vi "624WPI_DashboardGetInfo.vi"(7 "Vision":u16(ring) items=["Camera Off", "USB Camera SW", "USB Camera HW", "IP Camera"], 8 "Binding Refnum":refnum<notifier>, 9 "Window Mode Notifier":refnum<notifier>, 11 "TCP Cnx":refnum<k5>) -> (0 "Power and Errors":T2, 1 "Robot Metrics":T3, 2 "Status Info":T5, 3 "Control Info":T4 {"Team Station" items=["Red 1", "Red 2", "Red 3", "Blue 1", "Blue 2", "Blue 3"]}, 4 "Robot Mode":T1(ring), 5 "Process?":bool, 6 "Custom Dashboard Data":string)   [LabVIEW 2017]
uses:
  Dashboard Hijack Data.ctl
  <vilib>/Rock Robotics/WPI/Dashboard/WPI_DashboardLogging Global.vi
panel:
  out "port":u16
  # "CAN Metrics\nJS HID Outputs\nFree Mem"
  # "Need to merge in TCP info too"
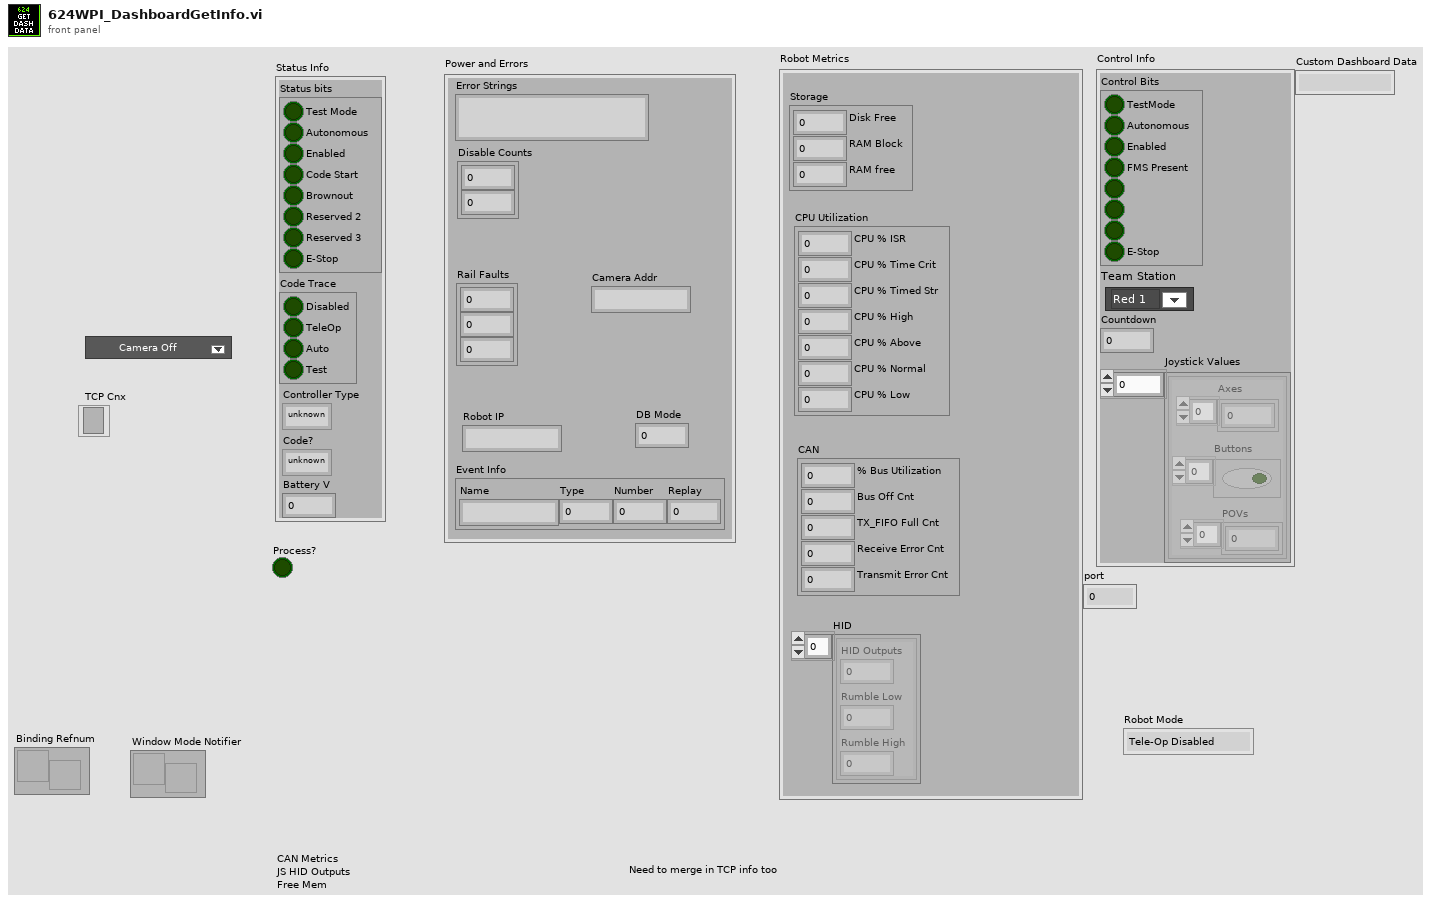
[diagram p1: front panel]
types:
  T1 = enum8{"Tele-Op Disabled", "Tele-Op Enabled", "Auto Disabled", "Auto Enabled", "Test Disabled", "Test Enabled", "Disconnected", "No Code", "E-Stop"}
  T2 = cluster{"Error Strings":string, "Disable Counts":cluster{u16, u16}, "Rail Faults":cluster{u16, u16, u16}, "Robot IP":string, "DB Mode":u8, "Event Info":cluster{"Name":string, "Type":u8, "Number":u16, "Replay":u8}, "Camera Addr":string}
  T3 = cluster{"Storage":cluster{"Disk Free":u64, "RAM Block":u32, "RAM free":u32}, "CPU Utilization":cluster{"CPU % ISR":sgl, "CPU % Time Crit":sgl, "CPU % Timed Str":sgl, "CPU % High":sgl, "CPU % Above":sgl, "CPU % Normal":sgl, "CPU % Low":sgl}, "CAN":cluster{"% Bus Utilization":sgl, "Bus Off Cnt":u32, "TX_FIFO Full Cnt":u32, "Receive Error Cnt":u8, "Transmit Error Cnt":u8}, "HID":cluster{"HID Outputs":u32, "Rumble Low":u16, "Rumble High":u16}[]}
  T4 = cluster{"Control Bits":cluster{"TestMode":bool, "Autonomous":bool, "Enabled":bool, "FMS Present":bool, bool, bool, bool, "E-Stop":bool}, "Team Station ":u8, "Countdown":sgl, "Joystick Values":cluster{"Axes":dbl[], "Buttons":bool[], "POVs":i16[]}[]}
  T5 = cluster{"Status bits":cluster{"Test Mode":bool, "Autonomous":bool, "Enabled":bool, "Code Start":bool, "Brownout":bool, "Reserved 2":bool, "Reserved 3":bool, "E-Stop":bool}, "Code Trace":cluster{"Disabled":bool, "TeleOp":bool, "Auto":bool, "Test":bool}, "Controller Type":enum16{"unknown", "cRIO", "roboRio"}, "Code?":enum16{"unknown", "noCode", "code"}, "Battery V":dbl}
  T6 = typedef "Dashboard Hijack Data.ctl" = cluster{"UDP Status string":string, "Extra data string":string}
  T7 = cluster{"TestMode":bool, "Autonomous":bool, "Enabled":bool, "FMS Present":bool, bool, bool, bool, "E-Stop":bool}
  T8 = enum16{"Standard", "Buffered", "CRLF", "Immediate"}
  T9 = cluster{"UDP Status":string, "TCP":string, "UDP Control":string}
  T10 = cluster{cluster{"Disk Free":u64, "RAM Block":u32, "RAM free":u32}, cluster{"CPU Load ISR":sgl, "CPU Load Time Critical Pr":sgl, "CPU Load Timed Str Pr":sgl, "CPU Load High Pr":sgl, "CPU Load Above Normal Pr":sgl, "CPU Load Normal Pr":sgl, "CPU Load Low Pr":sgl}, cluster{"% Bus Utilization":sgl, "Bus Off Cnt":u32, "TX_FIFO Full Cnt":u32, "Receive Error Cnt":u8, "Transmit Error Cnt":u8}, cluster{"HID Outputs":u32, "Rumble Low":u16, "Rumble High":u16}[]}
  T11 = cluster{"Status":cluster{"Test Mode":bool, "Autonomous":bool, "Enabled":bool, "Code Start":bool, "Brownout":bool, "Reserved 2":bool, "Reserved 3":bool, "E-Stop":bool}, cluster{bool, bool, bool, bool}, "ctrl":enum16{"unknown", "cRIO", "roboRio"}, "code?":enum16{"unknown", "noCode", "code"}, dbl}
  T12 = cluster{"Boolean array":cluster{"Boolean array[0]":bool, "Boolean array[1]":bool, "Boolean array[2]":bool, "Boolean array[3]":bool, "Boolean array[4]":bool, "Boolean array[5]":bool, "Boolean array[6]":bool, "Boolean array[7]":bool}, u8, "Countdown":sgl, cluster{dbl[], bool[], i16[]}[]}
  T13 = cluster{"Boolean array[0]":bool, "Boolean array[1]":bool, "Boolean array[2]":bool, "Boolean array[3]":bool, "Boolean array[4]":bool, "Boolean array[5]":bool, "Boolean array[6]":bool, "Boolean array[7]":bool}
  T14 = typedef "Protocol Operations.ctl" = enum16{"Unknown", "Keep Alive", "Client Hello", "Version not supported", "Server Hello Complete", "Assign", "Update", "No Op", "Server Hello", "Client Hello Complete", "Update Flags", "Delete Entry", "Delete All", "RPC Exec", "RPC Response"}
  T15 = typedef "Field Data.ctl" = cluster{"Dbl":dbl, "String":string, "Type":T16, "Boolean":bool, "Sequence #":T17, "Flags":u8}
  T16 = typedef "Field Type.ctl" = enum8{"Invalid", "Bool", "Numeric", "String", "Raw", "Boolean Array", "Numeric Array", "String Array", "RPC"}
  T17 = typedef "Sequence.ctl" = u16
  T18 = cluster{"Operation":T14, "Name":string, "Field Value":T15}[]
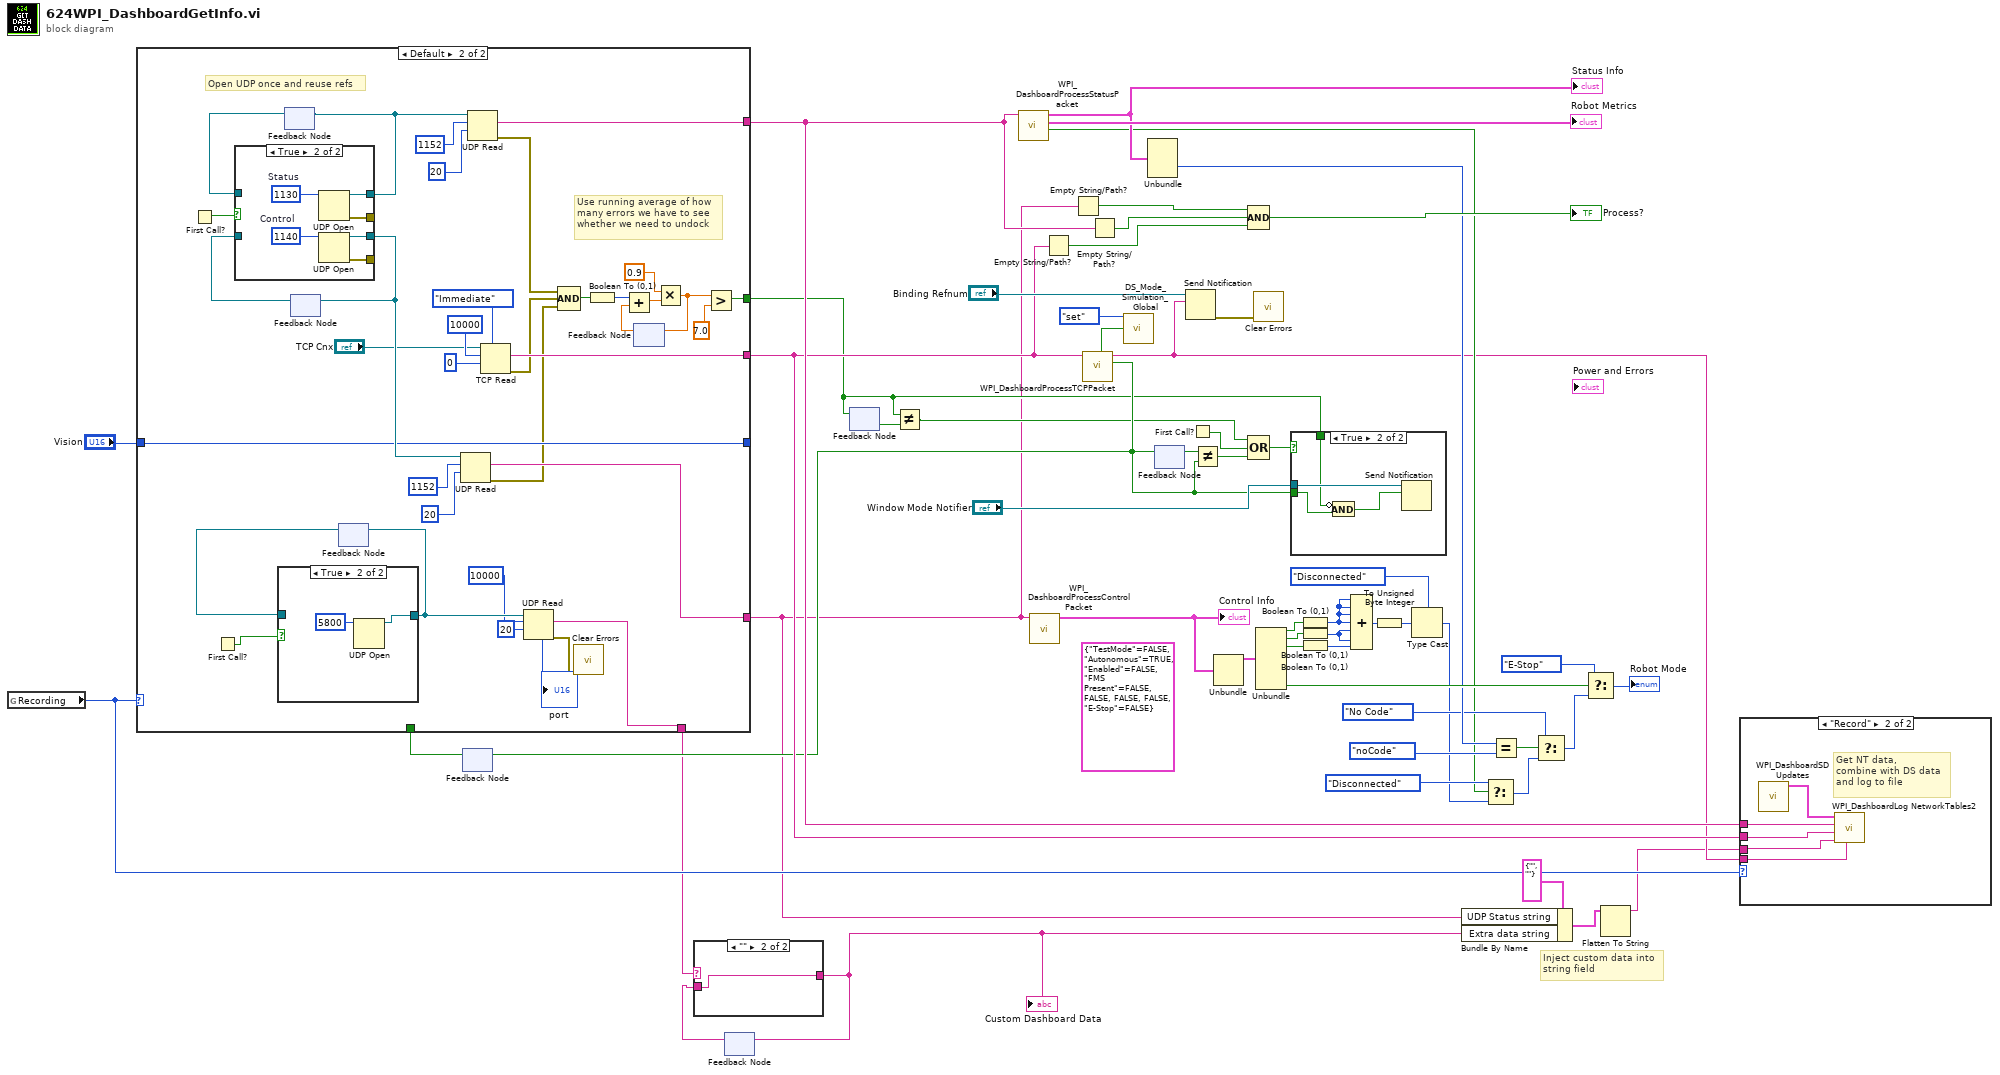
[diagram p0: block diagram]
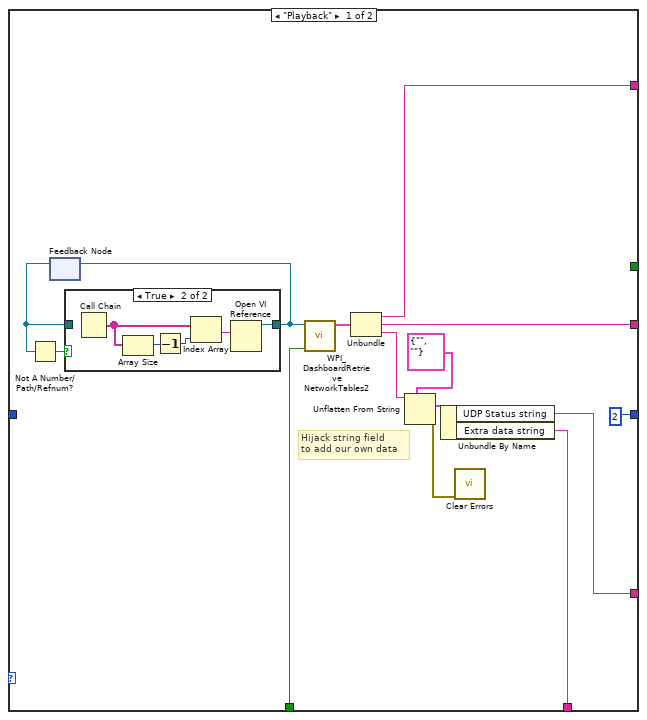
[diagram p4: hidden frame]
diagram:
  (unwired) T7 {"TestMode"=FALSE, "Autonomous"=TRUE, "Enabled"=FALSE, "FMS Present"=FALSE, FALSE, FALSE, FALSE, "E-Stop"=FALSE} ("Control Bits")
  # "Inject custom data into\nstring field"
  n1 = global read "WPI_DashboardLogging Global.vi" "Recording"() -> (w12:enum32{"Stop", "Record", "Playback"})
  n2 = feedback #1() -> (w14:bool)  [unwired: 1 in]
  n3 = case shown="Default" w12 {
    tunnel: [w58 w104] -> w7
    tunnel: [w65 w103] -> w18
    tunnel: [w64 w102] -> w17
    tunnel: w14 -> [w63 _]
    tunnel: "Vision" -> [_ w95]
    tunnel: [2 ("timeout ms (25000)") w95] -> _
    tunnel: [_ w84] -> w11
    tunnel: [w57 w83] -> w4
    frame "Playback" {
      # "Hijack string field\nto add our own data"
      n4 = feedback #2() -> (w69:refnum<vi>)  [unwired: 1 in]
      n5 = Not A Number/Path/Refnum?(number/path/refnum=w69) -> (NaN/Path/Refnum?=w68:bool)
      n6 = case shown="True" w68 {
        tunnel: w69 -> [w70 _]
        tunnel: [w70 w74] -> w66
        frame False {
        }
        frame True {
          n7 = Call Chain() -> (call chain=w73:string[])
          n8 = Array Size(array=w73) -> (size(s)=w72:i32)
          n9 = Decrement(x=w72) -> (x-1=w71:i32)
          n10 = Index Array(array=w73, index=w71) -> (element=w75:string)
          n11 = Open VI Reference(vi path=w75) -> (vi reference=w74:refnum<vi>)  [unwired: 5 in, 1 out]
        }
      }
      n12 = feedback-in #2(w66) -> ()
      n13 = call <vilib>:"WPI_DashboardRetrieve NetworkTables2.vi"("Docked Window"=w63, "DB Main Ref"=w66) -> ("Strings"=w67:T9)  [unwired: 9 in]
      n14 = Unbundle(w67) -> ("UDP Status"=w65:string, "TCP"=w64:string, "UDP Control"=w61:string)
      n15 = Unflatten From String(type=T6 {"UDP Status string"="", "Extra data string"=""} ("Dashboard Data Hijack"), binary string=w61) -> (value=w59:T6, error out=w56:errorcluster)  [unwired: 3 in, 1 out]
      n16 = Unbundle By Name(w59) -> ("UDP Status string"=w58:string, "Extra data string"=w57:string)
      n17 = call <vilib>:"Clear Errors.vi"("error in (no error)"=w56) -> ()  [unwired: 5 in, 2 out]
    }
    frame Default {
      # "Use running average of how\nmany errors we have to see\nwhether we need to undock"
      # "Open UDP once and reuse refs"
      n18 = First Call?() -> (First Call?: T/F=w101:bool)
      n19 = First Call?() -> (First Call?: T/F=w80:bool)
      n20 = feedback #3() -> (w99:refnum<k16>)  [unwired: 1 in]
      n21 = feedback #4() -> (w97:refnum<k16>)  [unwired: 1 in]
      n22 = case shown="True" w101 {
        tunnel: [w116 w120] -> w100
        tunnel: [_ w119] -> _
        tunnel: [w115 w118] -> w98
        tunnel: [_ w117] -> _
        tunnel: w99 -> [w116 _]
        tunnel: w97 -> [w115 _]
        frame False {
        }
        frame True {
          w121 = u16 1140  # Control
          w122 = u16 1130  # Status
          n23 = UDP Open(11:w122) -> (port=w120:refnum<k16>, 0:w119:errorcluster)  [unwired: 2 in, 3 out]
          n24 = UDP Open(11:w121) -> (port=w118:refnum<k16>, 0:w117:errorcluster)  [unwired: 2 in, 3 out]
        }
      }
      n25 = feedback-in #3(w100) -> ()
      n26 = feedback-in #4(w98) -> ()
      n27 = feedback #5() -> (w82:refnum<k16>)  [unwired: 1 in]
      n28 = case shown="True" w80 {
        tunnel: [w112 w113] -> w81
        tunnel: w82 -> [w112 _]
        frame False {
        }
        frame True {
          n29 = UDP Open(11:u16 5800 ("port")) -> (port=w113:refnum<k16>)  [unwired: 4 in, 2 out]
        }
      }
      n30 = feedback-in #5(w81) -> ()
      n31 = UDP Read(connection ID=w98, max size (548)=1152, timeout ms (25000)=20 ("length (rest)")) -> (data out=w104:string, error out=w92:errorcluster)  [unwired: 1 in, 3 out]
      n32 = UDP Read(connection ID=w100, max size (548)=1152, timeout ms (25000)=20 ("length (rest)")) -> (data out=w103:string, error out=w94:errorcluster)  [unwired: 1 in, 3 out]
      n33 = TCP Read(connection ID="TCP Cnx", bytes to read=10000 ("timeout ms (25000)"), 7:T8."Immediate" ("mode (standard)"), 9:0 ("timeout ms (25000)")) -> (data out=w102:string, error out=w93:errorcluster)  [unwired: 1 in, 1 out]
      n34 = UDP Read(connection ID=w81, max size (548)=10000, timeout ms (25000)=20) -> (data out=w83:string, error out=w78:errorcluster, 4:→"port":u16)  [unwired: 1 in, 2 out]
      n35 = Compound Arithmetic op=AND(w94, w93, w92) -> (w91:bool)
      n36 = call <vilib>:"Clear Errors.vi"("error in (no error)"=w78) -> ()  [unwired: 5 in, 2 out]
      n37 = Boolean To (0,1)(Boolean=w91) -> (0, 1=w90:i16)
      n38 = feedback #6() -> (w89:dbl)  [unwired: 1 in]
      n39 = Add(x=w90, y=w89) -> (x+y=w88:dbl)
      n40 = Multiply(x=0.9 ("timeout ms (25000)"), y=w88) -> (x*y=w86:dbl)
      n41 = feedback-in #6(w86) -> ()
      n42 = Greater?(x=w86, y=7.0 ("timeout ms (25000)")) -> (0:w84:bool)
    }
  }
  n43 = feedback #7() -> (w3:string)  [unwired: 1 in]
  n44 = case shown="\"\"" w4 {
    selector: w4 -> [w123 _]
    tunnel: [w123 w124] -> w2
    tunnel: w3 -> [_ w124]
    frame Default {
    }
    frame "" {
    }
  }
  "Custom Dashboard Data" <- w2
  n45 = feedback-in #7(w2) -> ()
  n46 = feedback #8() -> (w10:bool)  [unwired: 1 in]
  n47 = feedback-in #8(w11) -> ()
  n48 = Not Equal?(x=w11, y=w10) -> (x != y?=w9:bool)
  n49 = call <vilib>:"WPI_DashboardProcessStatusPacket.vi"("data in"=w18) -> ("Disconnected"=w21:bool, "Robot Metrics"=→"Robot Metrics":T10, "Status Cluster"=w35:T11)  [unwired: 8 in]
  "Status Info" <- w35
  n50 = call <vilib>:"WPI_DashboardProcessControlPacket.vi"("data in"=w7) -> ("Control Info"=w43:T12)  [unwired: 10 in]
  "Control Info" <- w43
  n51 = Empty String/Path?(string/path=w17) -> (empty?=w53:bool)
  n52 = Empty String/Path?(string/path=w7) -> (empty?=w51:bool)
  n53 = call <vilib>:"WPI_DashboardProcessTCPPacket.vi"("data in"=w17) -> ("Docked"=w15:bool, "Robot IP"=w16:string, "Simulated"=w19:bool)  [unwired: 6 in, 2 out]
  n54 = feedback-in #1(w15) -> ()
  n55 = Empty String/Path?(string/path=w18) -> (empty?=w52:bool)
  n56 = call <vilib>:"DS_Mode_Simulation_Global.vi"("menu"=enum16{"set", "get"}."set", "simulated? in"=w19) -> ()  [unwired: 12 in, 2 out]
  n57 = Unbundle(w35) -> ("code?"=w31:enum16{"unknown", "noCode", "code"})  [unwired: 4 out]
  n58 = feedback #9() -> (w46:bool)  [unwired: 1 in]
  n59 = feedback-in #9(w15) -> ()
  n60 = Send Notification(notification=w16, notifier="Binding Refnum") -> (error out=w1:errorcluster)  [unwired: 1 in, 1 out]
  n61 = First Call?() -> (First Call?: T/F=w48:bool)
  n62 = Not Equal?(x=w46, y=w15) -> (x != y?=w47:bool)
  n63 = Unbundle(w43) -> ("Boolean array"=w42:T13)  [unwired: 3 out]
  n64 = Compound Arithmetic op=AND(w51, w52, w53) -> (→"Process?":bool)
  n65 = Compound Arithmetic op=OR(w9, w48, w47) -> (w49:bool)
  n66 = call <vilib>:"Clear Errors.vi"("error in (no error)"=w1) -> ()  [unwired: 5 in, 2 out]
  n67 = Unbundle(w42) -> ("Boolean array[0]"=w37:bool, "Boolean array[1]"=w38:bool, "Boolean array[2]"=w40:bool, "Boolean array[7]"=w34:bool)  [unwired: 4 out]
  n68 = case shown="True" w49 {
    tunnel: "Window Mode Notifier" -> [_ w128]
    tunnel: w15 -> [_ w126]
    tunnel: w11 -> [_ w127]
    frame False {
    }
    frame True {
      n69 = Compound Arithmetic op=AND(invert w127, w126) -> (w125:bool)
      n70 = Send Notification(notification=w125, notifier=w128) -> ()  [unwired: 1 in, 2 out]
    }
  }
  n71 = Boolean To (0,1)(Boolean=w37) -> (0, 1=w36:i16)
  n72 = Boolean To (0,1)(Boolean=w38) -> (0, 1=w39:i16)
  n73 = Boolean To (0,1)(Boolean=w40) -> (0, 1=w41:i16)
  n74 = Compound Arithmetic op=ADD(w36, w36, w36, w36, w39, w39, w41) -> (w25:i16)
  n75 = To Unsigned Byte Integer(number=w25) -> (unsigned 8bit integer=w20:u8)
  n76 = Type Cast(type=T1."Disconnected" ("Mode"), x=w20) -> (*(type *) &x=w24:T1)
  n77 = Bundle By Name(cluster=T6 {"UDP Status string"="", "Extra data string"=""} ("Dashboard Data Hijack"), "UDP Status string"=w7, "Extra data string"=w2) -> (w6:T6)
  n78 = Select(t=T1."Disconnected" ("Mode"), s=w21, f=w24) -> (s? t:f=w27:T1)
  n79 = Equal?(x=w31, y=enum16{"unknown", "noCode", "code"}."noCode" ("code?")) -> (x = y?=w30:bool)
  n80 = Select(t=T1."No Code" ("Mode"), s=w30, f=w27) -> (s? t:f=w29:T1)
  n81 = Select(t=T1."E-Stop" ("Mode"), s=w34, f=w29) -> (s? t:f=→"Robot Mode":T1)
  n82 = Flatten To String(anything=w6) -> (data string=w5:string)  [unwired: 3 in, 2 out]
  n83 = case shown="\"Record\"" w12 {
    tunnel: w18 -> [_ w130]
    tunnel: w17 -> [_ w131]
    tunnel: w5 -> [_ w132]
    tunnel: w16 -> [_ w129]
    frame Default {
    }
    frame "Record" {
      # "Get NT data,\ncombine with DS data\nand log to file"
      n84 = call <vilib>:"WPI_DashboardSD Updates.vi"() -> ("Collected Data"=w133:T18)  [unwired: 11 in]
      n85 = call <vilib>:"WPI_DashboardLog NetworkTables2.vi"("Robot IP"=w129, "UDP Control"=w132, "TCP"=w131, "UDP Status"=w130, "NT Data Values"=w133) -> ()  [unwired: 7 in]
    }
  }
